vi "lum.vi"(8 "lum":dbl) -> (0 "JOUR/NUIT":string="Nuit")   [LabVIEW 2017]
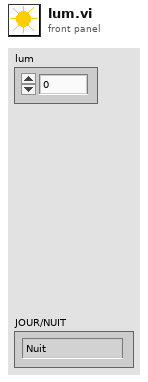
[diagram p1: front panel]
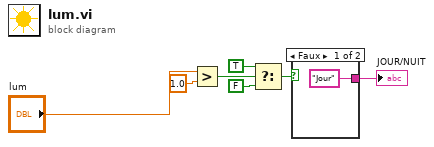
[diagram p0: block diagram]
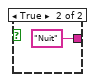
[diagram p2: hidden frame]
diagram:
  n1 = Greater?(x="lum", y=1.0) -> (0:w3:bool)
  n2 = Select(t=TRUE, s=w3, f=FALSE) -> (s? t:f=w5:bool)
  n3 = case shown="Faux" w5 {
    tunnel: ["Jour" "Nuit"] -> w4
    frame False {
    }
    frame True {
    }
  }
  "JOUR/NUIT" <- w4
